vi "Test_WriteValue_CheckText_TextUpdated.vi"(8 "error in (no error)":errorcluster, 11 "TestCase in":refnum<class "TestBooleanTextBinding.lvclass">) -> (0 "error out":errorcluster, 3 "TestCase out":refnum<class "TestBooleanTextBinding.lvclass">)   [LabVIEW 2017, in "TestBooleanTextBinding.lvclass"]
uses:
  TestBooleanTextBinding.lvclass
  Source/Concrete/BooleanTextBinding/BooleanTextBinding.lvclass/BooleanTextBinding.ctl
  Source/Concrete/BooleanTextBinding/BooleanTextBinding.lvclass
  C:/Git/composed-transport/Source/ITransport/ITransport.lvclass
  <vilib>/Utility/error.llb/Error Cluster From Error Code.vi
  Source/ITransport/ITransport.lvclass
panel:
  in  "OK Button":bool
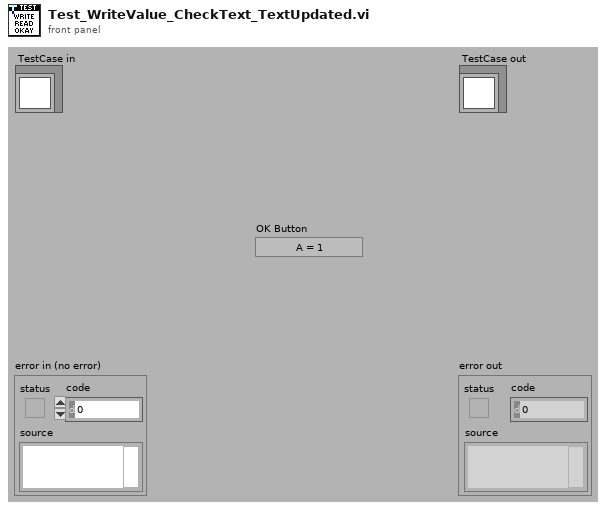
[diagram p1: front panel]
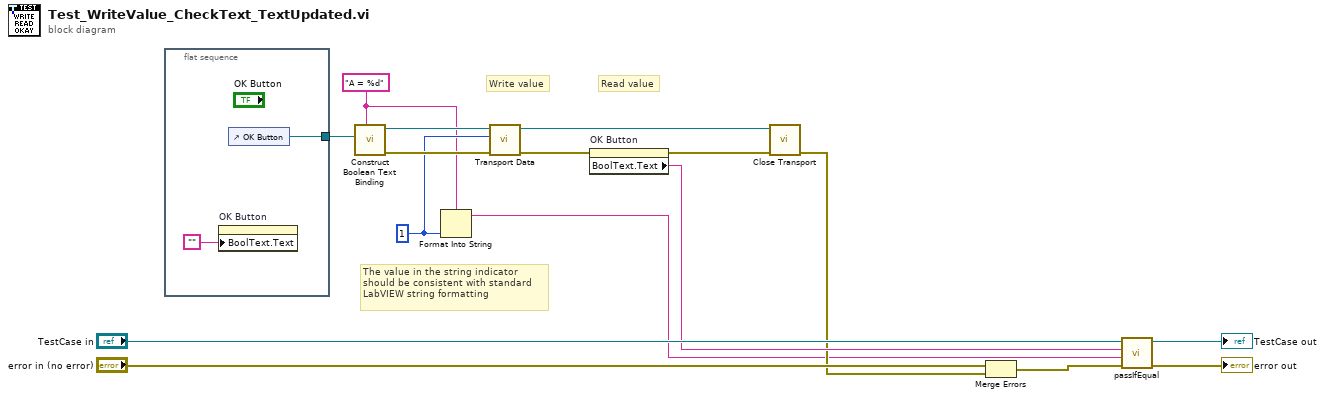
[diagram p0: block diagram]
diagram:
  w2 = "A = %d" ("Format String")
  w3 = 1
  # "The value in the string indicator\nshould be consistent with standard\nLabVIEW string formatting"
  # "Read value"
  # "Write value"
  n1 = flat-sequence {
    tunnel: [w18] -> w8
    frame #0 {
      n2 = property on="OK Button" class="Bool"("BoolText.Text"="") -> ()  [unwired: 2 in, 2 out]
      n3 = control-ref of="OK Button"() -> (w18:refnum<vi>)
    }
  }
  n4 = call "Construct Boolean Text Binding.vi"("Format String"=w2, "Bool Refnum"=w8) -> ("error out"=w10:errorcluster, "BooleanTextBinding"=w12:refnum<class "BooleanTextBinding.lvclass">)  [unwired: 8 in]
  n5 = Format Into String(format string=w2, w3) -> (resulting string=w1:string)  [unwired: 2 in, 1 out]
  n6 = call "Transport Data.vi"("error in (no error)"=w10, "Value"=w3, "ITransport in"=w12) -> ("error out"=w7:errorcluster, "ITransport out"=w9:refnum<class "BooleanTextBinding.lvclass">)  [unwired: 7 in]
  n7 = property on="OK Button" class="Bool"(error in=w7) -> (error out=w6:errorcluster, "BoolText.Text"=w5:string)  [unwired: 1 in, 1 out]
  n8 = call-dynamic "Close Transport.vi"("error in (no error)"=w6, "ITransport in"=w9) -> ("error out"=w4:errorcluster)  [unwired: 9 in]
  n9 = Merge Errors("error in (no error)", w4) -> (w11:errorcluster)
  n10 = call-dynamic "passIfEqual.vi"("error in (no error)"=w11, "y"=w1, "x"=w5, "TestCase in"="TestCase in") -> ("error out"=→"error out":errorcluster, "TestCase out"=→"TestCase out":refnum<class "TestBooleanTextBinding.lvclass">)  [unwired: 6 in]
